vi "PID append overwrite.vi"(6 "temperature":dbl, 7 "append/overwrite":enum16{"append", "overwrite"}(ring)=enum."overwrite", 8 "PID freq":dbl[](array[numeric])=[204.17553, 205.38327, 210.4933, 251.49092, 252.54665, 255.47144, 256.28856, 266.09474, 267.31354, 287.9551, 308.06888, 316.32045, 316.72441, 337.09714, 339.25692, 353.42129, 354.70138, 356.46473, 366.42846, 367.71161, 379.63344, 381.40641, 392.0567, 394.50308, 404.19029, 420.65746, 437.25062, 457.25667, 459.18248, 468.93997, 498.61795, 500.34276, 506.41857], 10 "ctl kind IN":T1, 11 "sweep folder":path) -> (3 "sweep folder out":path)   [LabVIEW 2015]
uses:
  ctl -- name dispatcher -- action.ctl
  next chunk read-write PID -- action.ctl
  array -- find index - real.vi
  array -- interpolate -- i.vi
  Q -- check range -- i -- real.vi
  Q - not nan -- real.vi
  file -- read list of lines.vi
  parse -- find first line.vi
  parse -- get list of matches -- numbers.vi
  <vilib>/Utility/file.llb/Write To Spreadsheet File.vi
  <vilib>/Utility/file.llb/Write To Spreadsheet File (string).vi
  <vilib>/gmath/function.llb/Binomial Coefficient.vi
panel:
  in  "freq PID file IN":string="ctl_PID_peak_DUMP.dat"
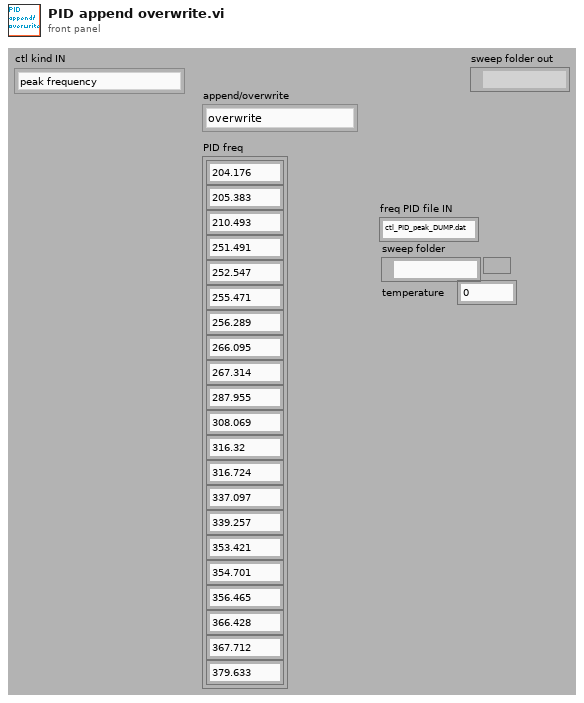
[diagram p1: front panel]
types:
  T1 = typedef "ctl -- name dispatcher -- action.ctl" = enum16{"peak frequency", "peak frequency DUMP", "peak gamma DUMP", "peak gamma", "peak frequency TEST", "peak gamma TEST", "ultrasonic power", "time in gamma", "set temperature ", "set temperature timer", "peak default gamma", "last scan file", "peak freq gamma TEST", "peak NAMES", "errors", "P_I_D", "P", "I", "D", "power vs time", "power vs time TIMER", "void", "power log", "set temperature - SINE", "itc ltc log", "peak - time in gamma"}
  T2 = typedef "next chunk read-write PID -- action.ctl" = enum16{"read", "interpolate", "append col", "write", "write PID col", "append PID col", "interpolate - bezier"}
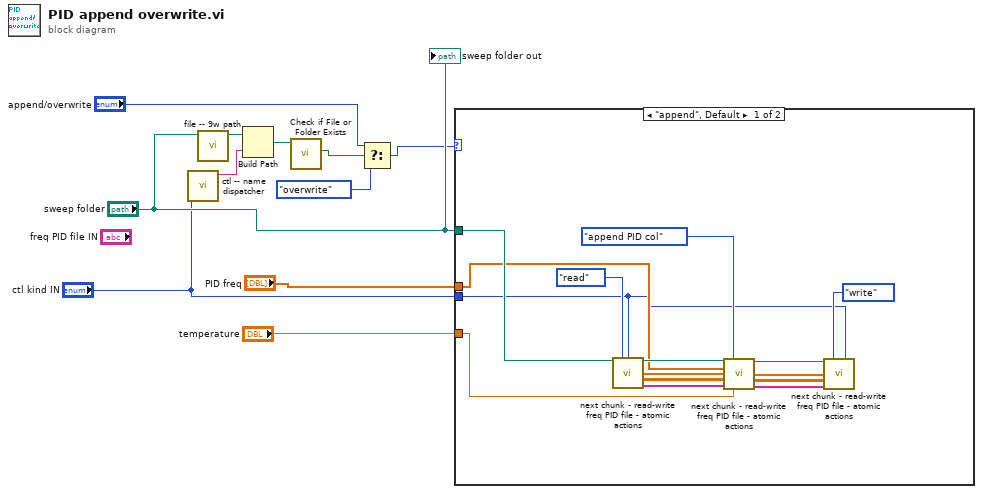
[diagram p0: block diagram]
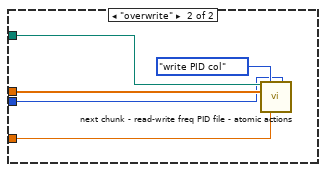
[diagram p2: hidden frame]
diagram:
  n1 = call "ctl -- name dispatcher.vi"("ctl name dispatch"="ctl kind IN") -> ("ctl file name"=w2:string)  [unwired: 8 in, 2 out]
  n2 = call "file -- 9w path.vi"("sweep folder"="sweep folder") -> ("9w path"=w10:path)  [unwired: 10 in]
  n3 = Build Path(base path=w10, name or relative path=w2) -> (appended path=w11:path)
  n4 = call <vilib>:"Check if File or Folder Exists.vi"("path"=w11) -> ("file or folder exists?"=w8:bool)  [unwired: 8 in, 2 out]
  n5 = Select(t="append/overwrite", s=w8, f=enum16{"append", "overwrite"}."overwrite") -> (s? t:f=w5:enum16{"append", "overwrite"})
  n6 = case shown="\"append\", Default" w5 {
    tunnel: "sweep folder" -> [w16 w30]
    tunnel: "PID freq" -> [w13 w29]
    tunnel: "temperature" -> [w14 w28]
    tunnel: "ctl kind IN" -> [w12 w27]
    frame "append", Default {
      n7 = call "next chunk - read-write freq PID file - atomic actions .vi"("sweep folder path"=w16, "PID action"=next_chunk_read-write_PID_--_action."read", "ctl kind IN"=w12) -> ("sweep folder path out"=w22:path, "temperatures"=w24:dbl[], "frequencies"=w25:dbl[][], "header"=w26:string[])  [unwired: 8 in, 1 out]
      n8 = call "next chunk - read-write freq PID file - atomic actions .vi"("sweep folder path"=w22, "PID action"=next_chunk_read-write_PID_--_action."append PID col", "PID freq IN"=w13, "temperatures IN"=w24, "frequencies IN"=w25, "header IN"=w26, "temperature"=w14) -> ("sweep folder path out"=w21:path, "temperatures"=w20:dbl[], "frequencies"=w19:dbl[][], "header"=w18:string[])  [unwired: 4 in, 1 out]
      n9 = call "next chunk - read-write freq PID file - atomic actions .vi"("sweep folder path"=w21, "PID action"=next_chunk_read-write_PID_--_action."write", "ctl kind OUT"=w12, "temperatures IN"=w20, "frequencies IN"=w19, "header IN"=w18) -> ()  [unwired: 5 in, 5 out]
    }
    frame "overwrite" {
      n10 = call "next chunk - read-write freq PID file - atomic actions .vi"("sweep folder path"=w30, "PID action"=next_chunk_read-write_PID_--_action."write PID col", "ctl kind OUT"=w27, "PID freq IN"=w29, "temperature"=w28) -> ()  [unwired: 6 in, 5 out]
    }
  }
  "sweep folder out" <- "sweep folder"
